vi "Decode_scancodes-onlylowercases_171213.vi"(4 "ScanCode":i16) -> (1 "String":string)   [LabVIEW 2016]
doc: "Decode scanscodes into ascii.vi takes the scancode, mods, and platmods to index a case structure that outputs the ASCII value and the numeric value of the ASCII. Use this VI in the key up event if you want to programatically capture keystrikes.\n\nThe VI is easy to use, but tedious to write. There are 93 cases, each of which was experimentally verified."
panel:
  # "Select Help»Show Context Help and move the cursor \nover the VI icon to display help for this VI."
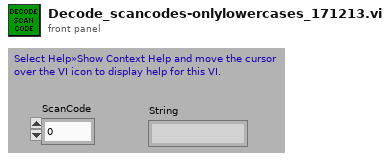
[diagram p1: front panel]
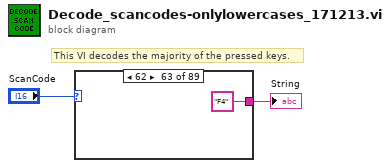
[diagram p0: block diagram]
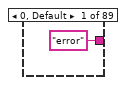
[diagram p2: hidden frame]
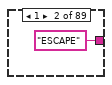
[diagram p3: hidden frame]
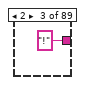
[diagram p4: hidden frame]
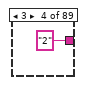
[diagram p5: hidden frame]
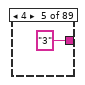
[diagram p6: hidden frame]
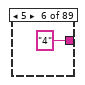
[diagram p7: hidden frame]
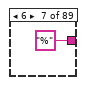
[diagram p8: hidden frame]
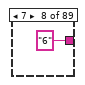
[diagram p9: hidden frame]
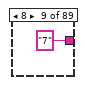
[diagram p10: hidden frame]
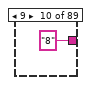
[diagram p11: hidden frame]
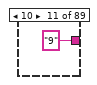
[diagram p12: hidden frame]
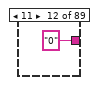
[diagram p13: hidden frame]
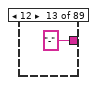
[diagram p14: hidden frame]
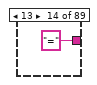
[diagram p15: hidden frame]
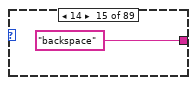
[diagram p16: hidden frame]
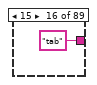
[diagram p17: hidden frame]
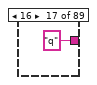
[diagram p18: hidden frame]
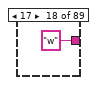
[diagram p19: hidden frame]
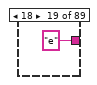
[diagram p20: hidden frame]
diagram:
  # "This VI decodes the majority of the pressed keys."
  n1 = case shown="62" "ScanCode" {
    tunnel: ["error" "ESCAPE" "!" "2" "3" "4" "%" "6" "7" "8" "9" "0" "-" "=" "backspace" "tab" "q" "w" "e" "r" "t" "y" "u" "i" "o" "p" "[" "}" "Enter" "control" "a" "s" "d" "f" "g" "h" "j" "k" "l" ";" "'" "`" "LSHIFT" ";" "z" "x" "c" "v" "b" "n" "m" "," "." "/" "RSHIFT" "/" "RSHIFT" "SPACE" "CAPSLOCK" "F1" "F2" "F3" "F4" "F5" "F6" "F7" "F8" "F9" "F10" "numlock" "error" "7" "UP" "9" "-" "4" "5" "6" "+" "END" "2" "PAGEDOWN" "0" "." "F11" "F12" "left win key" "right win key" "select"] -> w2
    frame 0, Default {
    }
    frame 1 {
    }
    frame 2 {
    }
    frame 3 {
    }
    frame 4 {
    }
    frame 5 {
    }
    frame 6 {
    }
    frame 7 {
    }
    frame 8 {
    }
    frame 9 {
    }
    frame 10 {
    }
    frame 11 {
    }
    frame 12 {
    }
    frame 13 {
    }
    frame 14 {
    }
    frame 15 {
    }
    frame 16 {
    }
    frame 17 {
    }
    frame 18 {
    }
    frame 19 {
    }
    frame 20 {
    }
    frame 21 {
    }
    frame 22 {
    }
    frame 23 {
    }
    frame 24 {
    }
    frame 25 {
    }
    frame 26 {
    }
    frame 27 {
    }
    frame 28 {
    }
    frame 29 {
    }
    frame 30 {
    }
    frame 31 {
    }
    frame 32 {
    }
    frame 33 {
    }
    frame 34 {
    }
    frame 35 {
    }
    frame 36 {
    }
    frame 37 {
    }
    frame 38 {
    }
    frame 39 {
    }
    frame 40 {
    }
    frame 41 {
    }
    frame 42 {
    }
    frame 43 {
    }
    frame 44 {
    }
    frame 45 {
    }
    frame 46 {
    }
    frame 47 {
    }
    frame 48 {
    }
    frame 49 {
    }
    frame 50 {
    }
    frame 51 {
    }
    frame 52 {
    }
    frame 53 {
    }
    frame 54 {
    }
    frame 55 {
    }
    frame 56 {
    }
    frame 57 {
    }
    frame 58 {
    }
    frame 59 {
    }
    frame 60 {
    }
    frame 61 {
    }
    frame 62 {
    }
    frame 63 {
    }
    frame 64 {
    }
    frame 65 {
    }
    frame 66 {
    }
    frame 67 {
    }
    frame 68 {
    }
    frame 69 {
    }
    frame 70 {
    }
    frame 71 {
    }
    frame 72 {
    }
    frame 73 {
    }
    frame 74 {
    }
    frame 75 {
    }
    frame 76 {
    }
    frame 77 {
    }
    frame 78 {
    }
    frame 79 {
    }
    frame 80 {
    }
    frame 81 {
    }
    frame 82 {
    }
    frame 83 {
    }
    frame 87 {
    }
    frame 88 {
    }
    frame 91 {
    }
    frame 92 {
    }
    frame 93 {
    }
  }
  "String" <- w2
